vi "_FileSync.Test.vi"() -> ()   [LabVIEW 2024, in "EQMF.lvlib" / "File Utils.lvlib"]
uses:
  File Utils.lvlib
  Sync/File.Sync Item Record.ctl
  Sync/File.Sync Item Log Record.ctl
  Sync/File.Sync.lvclass
panel:
  out "Elapsed":dbl
  out "Next Sync":dbl
  in  "Exit":bool
  in  "Sync Now":bool
  out "Event Log":T1[](array[typedef]) {"Last Sync" format="%<%I:%M:%S %p>T"}
  out "Sync Items":T2[](array[typedef])
  out "Sync Error":errorcluster
  out "Init Error":errorcluster
  in  "Config File":path
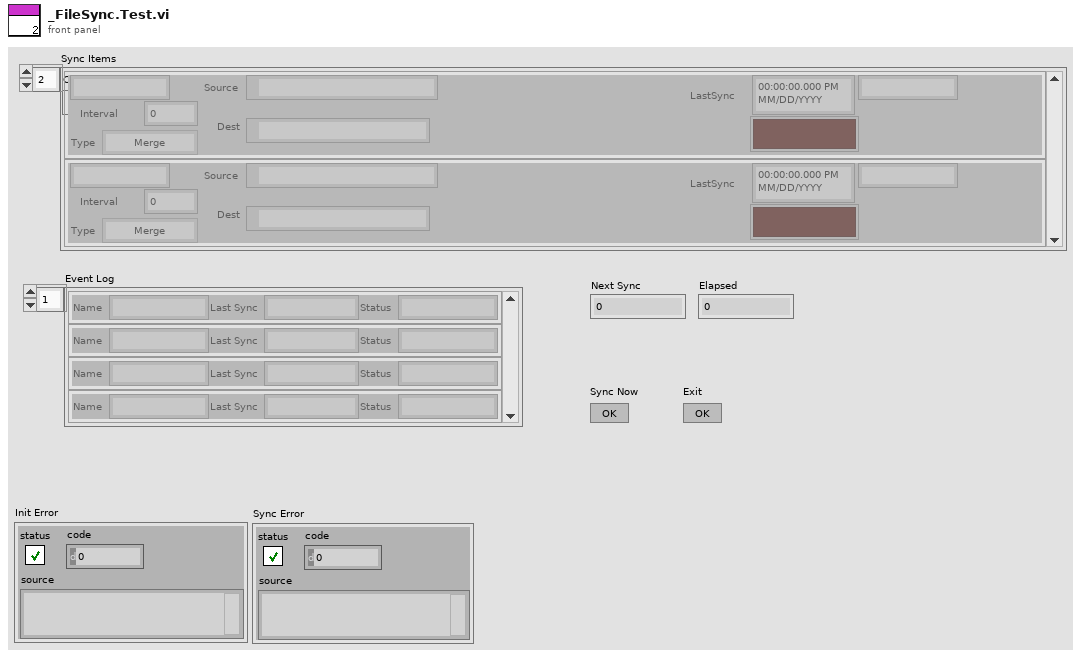
[diagram p1: front panel]
types:
  T1 = typedef "EQMF.lvlib/File Utils.lvlib/File.Sync.lvclass/File.Sync Item Log Record.ctl" = cluster{"Name":string, "Last Sync":timestamp, "Status":string}
  T2 = typedef "EQMF.lvlib/File Utils.lvlib/File.Sync.lvclass/File.Sync Item Record.ctl" = cluster{"Name":string, "Interval":dbl, "Source":path, "Dest":path, "LastSync":timestamp, "Status":string, "Error":bool, "Type":enum16{"Merge", "Match"}}
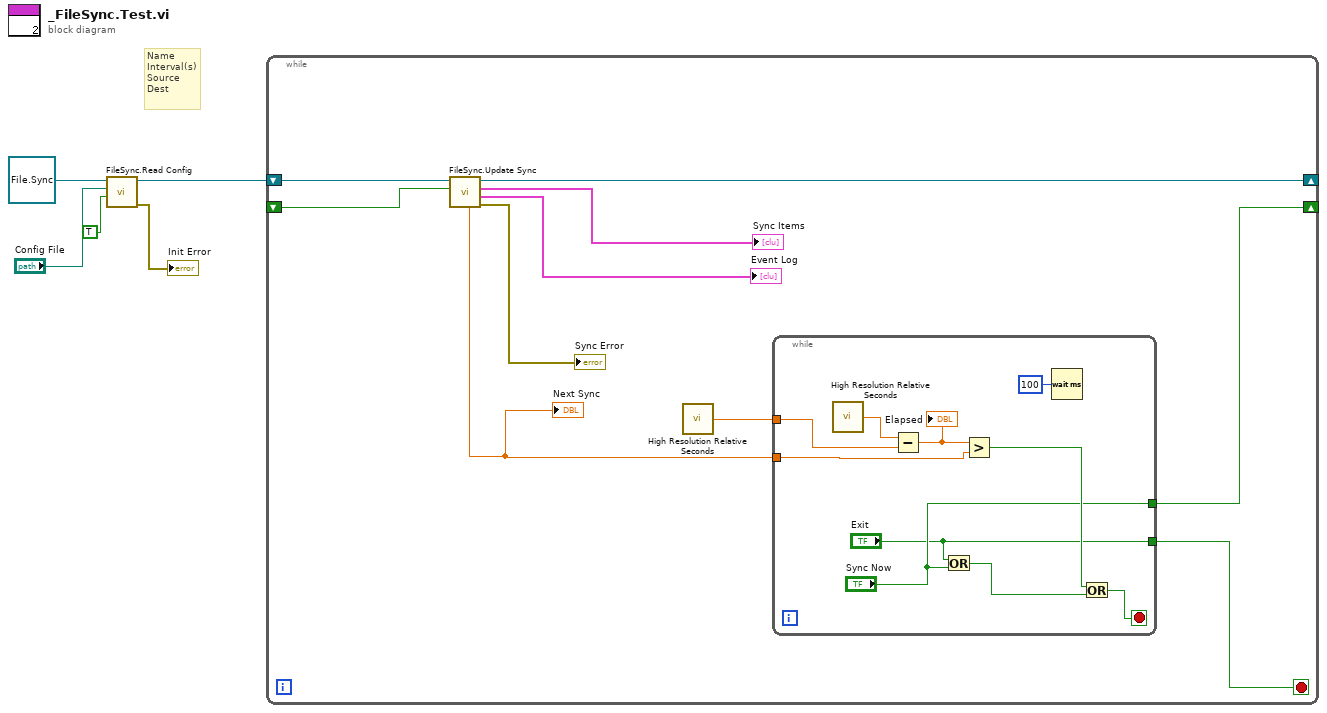
[diagram p0: block diagram]
diagram:
  # "Name\nInterval(s)\nSource\nDest"
  n1 = call-dynamic "FileSync.Read Config.vi"("Dialog"=TRUE, "Config File"="Config File", "File.Sync in"=refnum<class "File.Sync.lvclass"> refnum) -> ("error out"=→"Init Error":errorcluster, "File.Sync out"=w4:refnum<class "File.Sync.lvclass">)  [unwired: 5 in, 2 out]
  n2 = while {
    shift-right: [w11] -> _
    shift-left: w4 -> [w15]
    shift-right: [w8] -> _
    shift-left: _ -> [w7]
    stop <- w6 stop-if-true
    n3 = call-dynamic "FileSync.Update Sync.vi"("Normal(F)/Force Sync(T)"=w7, "File.Sync in"=w15) -> ("error out"=→"Sync Error":errorcluster, "Event Log"=→"Event Log":T1[], "Sync Items"=→"Sync Items":T2[], "File.Sync out"=w11:refnum<class "File.Sync.lvclass">, "Next Sync"=w10:dbl)  [unwired: 5 in]
    "Next Sync" <- w10
    n4 = call <vilib>:"High Resolution Relative Seconds.vi"() -> ("relative seconds"=w9:dbl)
    n5 = while {
      tunnel: w10 -> [w23]
      tunnel: w9 -> [w24]
      tunnel: ["Sync Now"] -> w8
      tunnel: ["Exit"] -> w6
      stop <- w21 stop-if-true
      n6 = call <vilib>:"High Resolution Relative Seconds.vi"() -> ("relative seconds"=w25:dbl)
      n7 = Subtract(x=w25, y=w24) -> (x-y=w16:dbl)
      "Elapsed" <- w16
      n8 = Or(x="Exit", y="Sync Now") -> (x .or. y?=w22:bool)
      n9 = Greater?(x=w16, y=w23) -> (0:w20:bool)
      n10 = Wait (ms)(milliseconds to wait=u32 100) -> ()  [unwired: 1 out]
      n11 = Or(x=w20, y=w22) -> (x .or. y?=w21:bool)
    }
  }
